vi "Enable Output.vi"(7 "Enable Output (T: Enable)":bool=TRUE, 8 "error in (no error)":errorcluster, 10 "Channel (0: Channel 1)":T1 items=["Channel 1", "Channel 2"], 11 "VISA resource name":refnum<visa-resource-name>) -> (0 "error out":errorcluster, 3 "VISA resource name out":refnum<visa-resource-name>)   [LabVIEW 2015, in "Tektronix AFG 3000 Series.lvlib"]
doc: "Enables or disables the output connector."
uses:
  Tektronix AFG 3000 Series.lvlib
  controls.llb/Channel.ctl
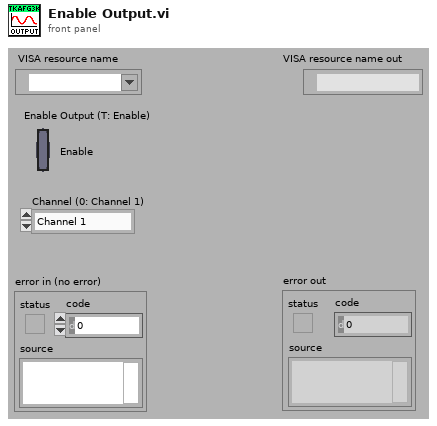
[diagram p1: front panel]
types:
  T1 = typedef "Channel.ctl" = u16
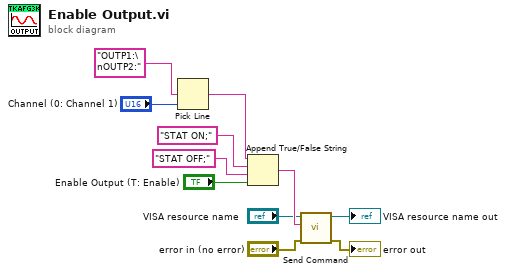
[diagram p0: block diagram]
diagram:
  n1 = Pick Line(multi-line string="OUTP1:\nOUTP2:" ("string (\"\")"), line index="Channel (0: Channel 1)") -> (output string=w6:string)  [unwired: 1 out]
  n2 = Append True/False String(1:"Enable Output (T: Enable)", 2:"STAT OFF;" ("true string"), 3:"STAT ON;" ("true string"), 4:w6) -> (0:w5:string)
  n3 = call "Send Command.vi"("error in (no error)"="error in (no error)", "write buffer"=w5, "VISA resource name"="VISA resource name") -> ("error out"=→"error out":errorcluster, "VISA resource name out"=→"VISA resource name out":refnum<visa-resource-name>)  [unwired: 7 out]
